vi "Multiclamp Init.vi"(5 "Gain":u16(ring)=1 items=["1"=1, "2"=2, "5"=5, "10"=10, "20"=20, "50"=50, "100"=100, "200"=200, "500"=500, "1000"=1000, "2000"=2000], 7 "Primary Output":u16(ring) items=["Vclamp - Membrane Current [0,5V/nA]", "Vclamp - Membrane Potential [10mV/10mV]", "Vclamp - Pipette Potential [1mV/mV]", "Vclamp - 100x AC Membrane Potential  [100mV/mV]", "Vclamp - External Command Potential  [50mV/mV]", "Vclamp - Auxiliary 1 Potential  [10mV/mV]", "Vclamp - Auxiliary 2 Current  [0,01V/nA]", "Iclamp - Membrane Potential  [10mV/mV]", "Iclamp - Membran Current  [0,5V/nA]", "Iclamp - Command Current  [0,5V/nA]", "Iclamp - 100x AC Membrane Potential  [100mV/mV]", "Iclamp - External Command Current [2,5V/nA]", "Iclamp - Auxiliary 1 Potential   [10mV/mV]", "Iclamp - Auxiliary 2 Current   [0,01V/nA]"], 8 "error in (no error)":errorcluster, 10 "Channel":u16(ring) items=["Channel 1", "Channel 2"], 11 "pszSerialNum":string="00106392") -> (0 "error out":errorcluster, 1 "pnError out":i32, 3 "Handler":i32)   [LabVIEW 2012, in "MultiClamp 700B Controls.lvlib"]
uses:
  MultiClamp 700B Controls.lvlib
  AxMultiClampMsg/AxMultiClampMsg.lvlib
panel:
  in  "Tab Control":enum32{"Page 1", "Page 2"}(tab)
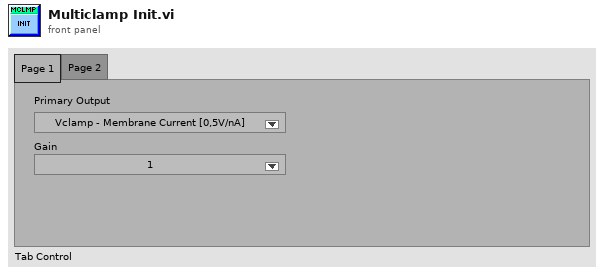
[diagram p1: front panel]
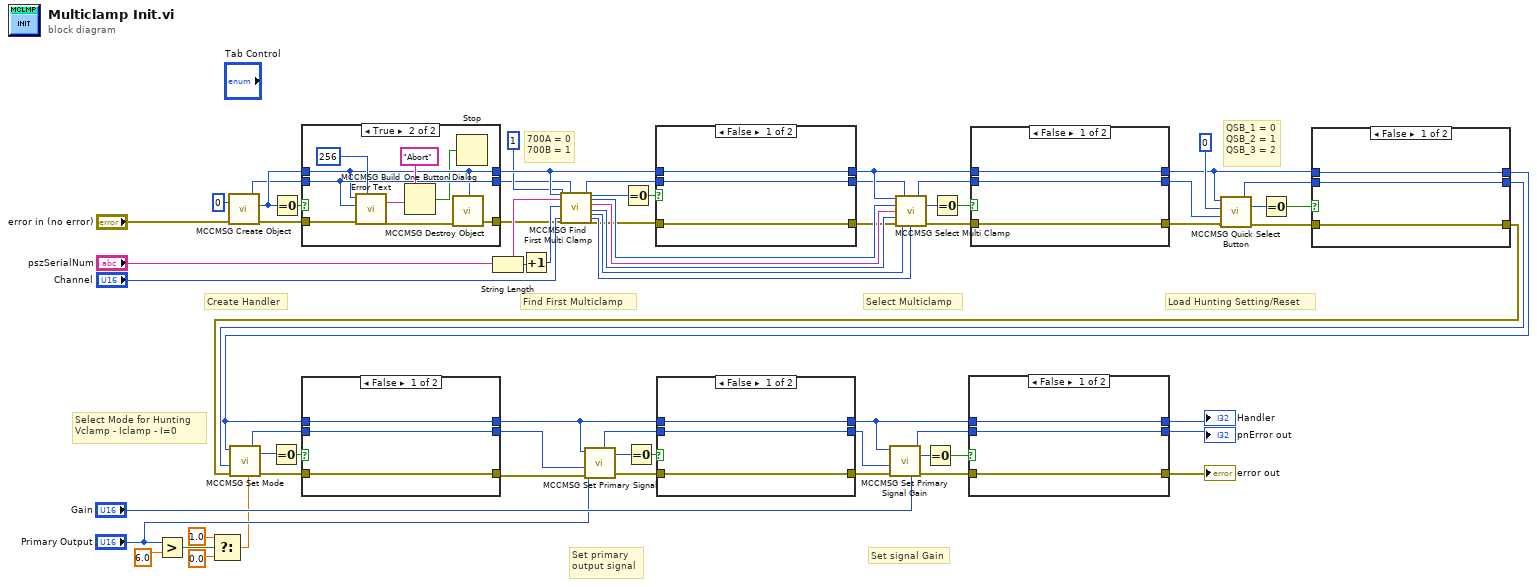
[diagram p0: block diagram]
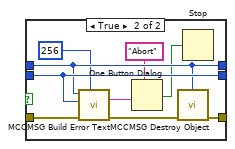
[diagram p2: hidden frame]
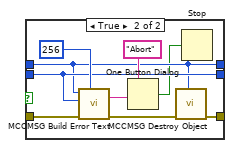
[diagram p3: hidden frame]
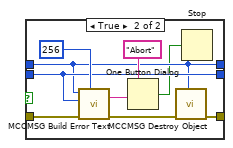
[diagram p4: hidden frame]
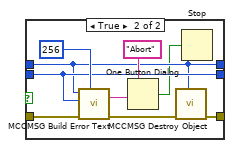
[diagram p5: hidden frame]
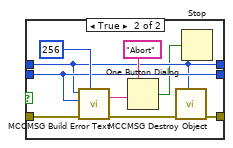
[diagram p6: hidden frame]
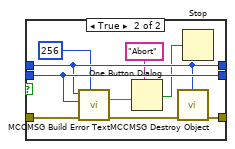
[diagram p7: hidden frame]
diagram:
  # "Set signal Gain"
  # "Set primary\noutput signal"
  # "Load Hunting Setting/Reset"
  # "QSB_1 = 0\nQSB_2 = 1\nQSB_3 = 2"
  # "Select Mode for Hunting\nVclamp - Iclamp - I=0"
  # "Select Multiclamp"
  # "Find First Multiclamp"
  # "Create Handler"
  # "700A = 0\n700B = 1"
  n1 = Greater?(x="Primary Output", y=6.0) -> (0:w5:bool)
  n2 = Select(t=1.0, s=w5, f=0.0) -> (s? t:f=w6:dbl)
  n3 = call "MCCMSG Create Object.vi"("error in (no error)"="error in (no error)", "pnError"=0) -> ("error out"=w14:errorcluster, "function return"=w15:i32, "pnError out"=w13:i32)  [unwired: 7 in]
  n4 = Equal To 0?(x=w15) -> (x = 0?=w12:bool)
  n5 = case shown="True" w12 {
    tunnel: w13 -> [w72 w77]
    tunnel: w14 -> [w70 w81]
    tunnel: w15 -> [w71 w74]
    tunnel: [w72 w77] -> w16
    tunnel: [w71 w74] -> w31
    tunnel: [w70 w76] -> w17
    frame False {
    }
    frame True {
      n6 = call "MCCMSG Build Error Text.vi"("uMaxLen"=u32 256, "error in (no error)"=w81, "nErrorNum"=w77, "hMCCmsg"=w74) -> ("error out"=w75:errorcluster, "sTxtBuf out"=w80:string)  [unwired: 5 in, 1 out]
      n7 = One Button Dialog(message=w80, button name ("OK")="Abort") -> (true=w73:bool)
      n8 = call "MCCMSG Destroy Object.vi"("error in (no error)"=w75, "hMCCmsg"=w74) -> ("error out"=w76:errorcluster)  [unwired: 9 in]
      n9 = Stop(stop? (T)=w73) -> ()
    }
  }
  n10 = String Length(string="pszSerialNum") -> (length=w29:i32)
  n11 = Increment(x=w29) -> (x+1=w40:i32)
  n12 = call "MCCMSG Find First Multi Clamp.vi"("hMCCmsg"=w31, "puModel"=u32 1, "pszSerialNum"="pszSerialNum", "uBufSize"=w40, "puChannelID"="Channel", "error in (no error)"=w17, "pnError"=w16) -> ("pnError out"=w22:i32, "function return"=w21:i32, "puModel out"=w37:u32, "pszSerialNum out"=w36:string, "puCOMPortID out"=w35:u32, "puDeviceID out"=w34:u32, "puChannelID out"=w33:u32, "error out"=w19:errorcluster)  [unwired: 13 in]
  n13 = Equal To 0?(x=w21) -> (x = 0?=w18:bool)
  n14 = case shown="False" w18 {
    tunnel: w22 -> [w84 w92]
    tunnel: w19 -> [w82 w93]
    tunnel: w31 -> [w83 w89]
    tunnel: [w84 w92] -> w23
    tunnel: [w83 w89] -> w30
    tunnel: [w82 w91] -> w20
    frame False {
    }
    frame True {
      n15 = call "MCCMSG Build Error Text.vi"("uMaxLen"=u32 256, "error in (no error)"=w93, "nErrorNum"=w92, "hMCCmsg"=w89) -> ("error out"=w90:errorcluster, "sTxtBuf out"=w88:string)  [unwired: 5 in, 1 out]
      n16 = One Button Dialog(message=w88, button name ("OK")="Abort") -> (true=w86:bool)
      n17 = call "MCCMSG Destroy Object.vi"("error in (no error)"=w90, "hMCCmsg"=w89) -> ("error out"=w91:errorcluster)  [unwired: 9 in]
      n18 = Stop(stop? (T)=w86) -> ()
    }
  }
  n19 = call "MCCMSG Select Multi Clamp.vi"("hMCCmsg"=w30, "uDeviceID"=w34, "pnError"=w23, "uModel"=w37, "pszSerialNum"=w36, "uCOMPortID"=w35, "error in (no error)"=w20, "uChannelID"=w33) -> ("pnError out"=w26:i32, "function return"=w25:i32, "error out"=w24:errorcluster)  [unwired: 4 in, 1 out]
  n20 = Equal To 0?(x=w25) -> (x = 0?=w28:bool)
  n21 = case shown="False" w28 {
    tunnel: w26 -> [w96 w101]
    tunnel: w24 -> [w94 w105]
    tunnel: w30 -> [w95 w98]
    tunnel: [w96 w101] -> w51
    tunnel: [w95 w98] -> w52
    tunnel: [w94 w99] -> w50
    frame False {
    }
    frame True {
      n22 = call "MCCMSG Build Error Text.vi"("uMaxLen"=u32 256, "error in (no error)"=w105, "nErrorNum"=w101, "hMCCmsg"=w98) -> ("error out"=w100:errorcluster, "sTxtBuf out"=w104:string)  [unwired: 5 in, 1 out]
      n23 = One Button Dialog(message=w104, button name ("OK")="Abort") -> (true=w97:bool)
      n24 = call "MCCMSG Destroy Object.vi"("error in (no error)"=w100, "hMCCmsg"=w98) -> ("error out"=w99:errorcluster)  [unwired: 9 in]
      n25 = Stop(stop? (T)=w97) -> ()
    }
  }
  n26 = call "MCCMSG Quick Select Button.vi"("error in (no error)"=w50, "pnError"=w51, "uButtonID"=u32 0, "hMCCmsg"=w52) -> ("error out"=w47:errorcluster, "pnError out"=w48:i32, "function return"=w49:i32)  [unwired: 5 in]
  n27 = Equal To 0?(x=w49) -> (x = 0?=w41:bool)
  n28 = case shown="False" w41 {
    tunnel: w48 -> [w108 w113]
    tunnel: w47 -> [w106 w117]
    tunnel: w52 -> [w107 w110]
    tunnel: [w108 w113] -> w46
    tunnel: [w107 w110] -> w45
    tunnel: [w106 w111] -> w54
    frame False {
    }
    frame True {
      n29 = call "MCCMSG Build Error Text.vi"("uMaxLen"=u32 256, "error in (no error)"=w117, "nErrorNum"=w113, "hMCCmsg"=w110) -> ("error out"=w112:errorcluster, "sTxtBuf out"=w116:string)  [unwired: 5 in, 1 out]
      n30 = One Button Dialog(message=w116, button name ("OK")="Abort") -> (true=w109:bool)
      n31 = call "MCCMSG Destroy Object.vi"("error in (no error)"=w112, "hMCCmsg"=w110) -> ("error out"=w111:errorcluster)  [unwired: 9 in]
      n32 = Stop(stop? (T)=w109) -> ()
    }
  }
  n33 = call "MCCMSG Set Mode.vi"("error in (no error)"=w54, "pnError"=w46, "uModeID"=w6, "hMCCmsg"=w45) -> ("error out"=w42:errorcluster, "pnError out"=w44:i32, "function return"=w43:i32)  [unwired: 5 in]
  n34 = Equal To 0?(x=w43) -> (x = 0?=w32:bool)
  n35 = case shown="False" w32 {
    tunnel: w44 -> [w120 w125]
    tunnel: w42 -> [w118 w129]
    tunnel: w45 -> [w119 w122]
    tunnel: [w120 w125] -> w2
    tunnel: [w119 w122] -> w3
    tunnel: [w118 w123] -> w4
    frame False {
    }
    frame True {
      n36 = call "MCCMSG Build Error Text.vi"("uMaxLen"=u32 256, "error in (no error)"=w129, "nErrorNum"=w125, "hMCCmsg"=w122) -> ("error out"=w124:errorcluster, "sTxtBuf out"=w128:string)  [unwired: 5 in, 1 out]
      n37 = One Button Dialog(message=w128, button name ("OK")="Abort") -> (true=w121:bool)
      n38 = call "MCCMSG Destroy Object.vi"("error in (no error)"=w124, "hMCCmsg"=w122) -> ("error out"=w123:errorcluster)  [unwired: 9 in]
      n39 = Stop(stop? (T)=w121) -> ()
    }
  }
  n40 = call "MCCMSG Set Primary Signal.vi"("error in (no error)"=w4, "pnError"=w2, "uSignalID"="Primary Output", "hMCCmsg"=w3) -> ("error out"=w58:errorcluster, "pnError out"=w60:i32, "function return"=w59:i32)  [unwired: 5 in]
  n41 = Equal To 0?(x=w59) -> (x = 0?=w56:bool)
  n42 = case shown="False" w56 {
    tunnel: w60 -> [w132 w137]
    tunnel: w58 -> [w130 w141]
    tunnel: w3 -> [w131 w134]
    tunnel: [w132 w137] -> w66
    tunnel: [w131 w134] -> w65
    tunnel: [w130 w135] -> w61
    frame False {
    }
    frame True {
      n43 = call "MCCMSG Build Error Text.vi"("uMaxLen"=u32 256, "error in (no error)"=w141, "nErrorNum"=w137, "hMCCmsg"=w134) -> ("error out"=w136:errorcluster, "sTxtBuf out"=w140:string)  [unwired: 5 in, 1 out]
      n44 = One Button Dialog(message=w140, button name ("OK")="Abort") -> (true=w133:bool)
      n45 = call "MCCMSG Destroy Object.vi"("error in (no error)"=w136, "hMCCmsg"=w134) -> ("error out"=w135:errorcluster)  [unwired: 9 in]
      n46 = Stop(stop? (T)=w133) -> ()
    }
  }
  n47 = call "MCCMSG Set Primary Signal Gain.vi"("error in (no error)"=w61, "pnError"=w66, "dGain"="Gain", "hMCCmsg"=w65) -> ("error out"=w62:errorcluster, "pnError out"=w64:i32, "function return"=w63:i32)  [unwired: 5 in]
  n48 = Equal To 0?(x=w63) -> (x = 0?=w57:bool)
  n49 = case shown="False" w57 {
    tunnel: w64 -> [w144 w152]
    tunnel: w62 -> [w142 w153]
    tunnel: w65 -> [w143 w149]
    tunnel: [w144 w152] -> w1
    tunnel: [w143 w149] -> w67
    tunnel: [w142 w151] -> w68
    frame False {
    }
    frame True {
      n50 = call "MCCMSG Build Error Text.vi"("uMaxLen"=u32 256, "error in (no error)"=w153, "nErrorNum"=w152, "hMCCmsg"=w149) -> ("error out"=w150:errorcluster, "sTxtBuf out"=w148:string)  [unwired: 5 in, 1 out]
      n51 = One Button Dialog(message=w148, button name ("OK")="Abort") -> (true=w146:bool)
      n52 = call "MCCMSG Destroy Object.vi"("error in (no error)"=w150, "hMCCmsg"=w149) -> ("error out"=w151:errorcluster)  [unwired: 9 in]
      n53 = Stop(stop? (T)=w146) -> ()
    }
  }
  "Handler" <- w67
  "error out" <- w68
  "pnError out" <- w1
